vi "Tikhonov's regularization.vi"(1 "Ordem":i32) -> (0 "Matriz de regularização":dbl[][](array[numeric]))   [LabVIEW 2018]
uses:
  <vilib>/Analysis/baseanly.llb/Real A x B.vi
  <vilib>/Analysis/NI_AALBase.lvlib
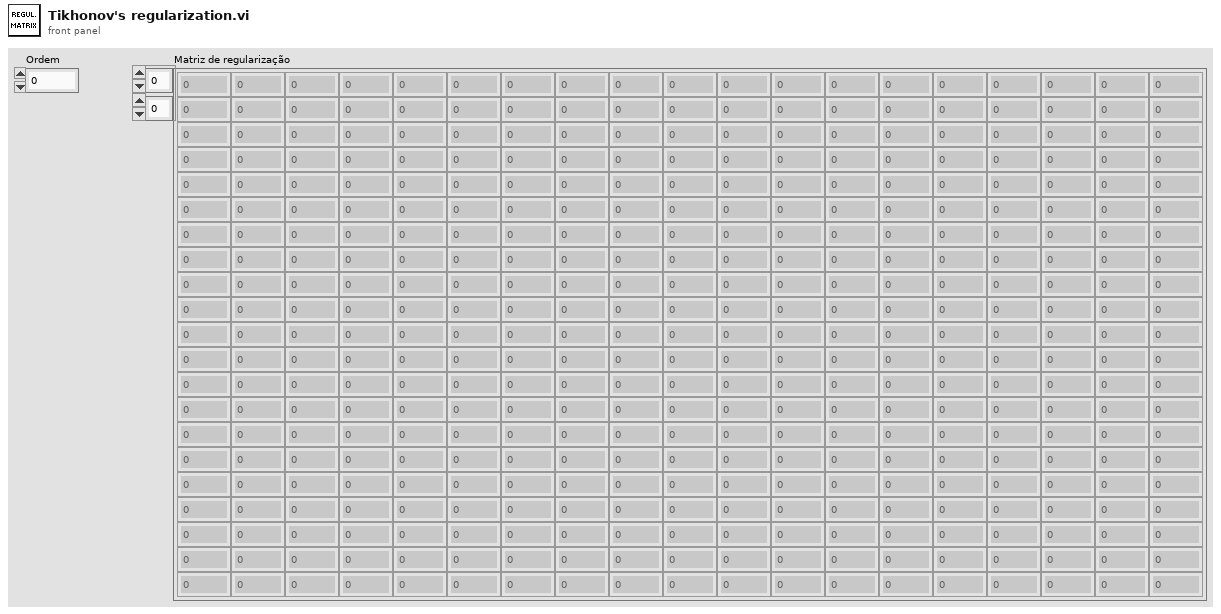
[diagram p1: front panel]
types:
  T1 = typedef "NI_Matrix.lvlib/RealMatrix.ctl" = dbl[][]
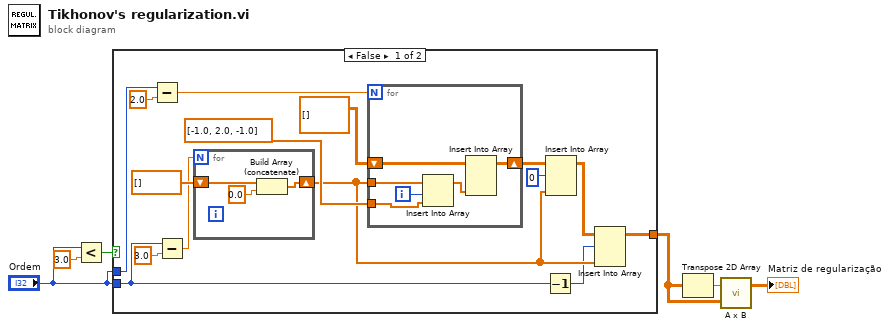
[diagram p0: block diagram]
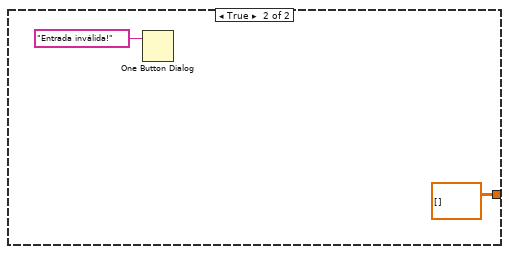
[diagram p2: hidden frame]
diagram:
  n1 = Less?(x="Ordem", y=3.0) -> (x < y?=w6:bool)
  n2 = case shown="False" w6 {
    tunnel: "Ordem" -> [w18 _]
    tunnel: [w11 dbl[][] [] ("2D array")] -> w1
    tunnel: "Ordem" -> [w8 _]
    frame False {
      n3 = Subtract(x=w18, y=2.0) -> (x-y=w17:dbl)
      n4 = Subtract(x=w8, y=3.0) -> (x-y=w7:dbl)
      n5 = for {
        N: w7 -> [_]
        shift-right: [w24] -> w12
        shift-left: dbl[] [] -> [w22]
        n6 = Build Array (concatenate)(w22, 0.0 ("element")) -> (w24:dbl[])
      }
      n7 = for {
        N: w17 -> [_]
        tunnel: dbl[] [-1.0, 2.0, -1.0] ("array") -> [w30]
        shift-right: [w27] -> w15
        shift-left: dbl[][] [] ("2D array") -> [w26]
        tunnel: w12 -> [w25]
        i -> [w29]
        n8 = Insert Into Array(array=w25, index=w29, new element=w30) -> (w28:dbl[])
        n9 = Insert Into Array(array=w26, new element=w28) -> (w27:dbl[][])  [unwired: 2 in]
      }
      n10 = Decrement(x=w8) -> (x-1=w10:i32)
      n11 = Insert Into Array(array=w15, index (row)=0, new element=w12) -> (w13:dbl[][])  [unwired: 1 in]
      n12 = Insert Into Array(array=w13, index (row)=w10, new element=w12) -> (w11:dbl[][])  [unwired: 1 in]
    }
    frame True {
      n13 = One Button Dialog(message="Entrada inválida!") -> ()  [unwired: 1 in, 1 out]
    }
  }
  n14 = Transpose 2D Array(2D array=w1) -> (transposed array=w2:dbl[][])
  n15 = call-poly <vilib>:"A x B.vi"("B"=w1, "A"=w2) -> ("A x B"=→"Matriz de regularização":T1)  [unwired: 1 out]
